vi "MAC BEG.vi"(0 "System no.":i32=1 min=1 max=4 step=1, 2 "Macro name":string, 5 "error in":errorcluster) -> (19 "error out":errorcluster)   [LabVIEW 2026]
doc: "Begin macro recording. Because controller will not answer VI queries during macro recording phase, command VIs cannot be run after this VI to define the macro. Run Define macro contents.vi and finish with MAC END.vi to define a macro.\n\nC-702, C-848, C-867, C-877, C-880, C-884, C-886, C-887, C-891, E-516, E-517, E-518, E-727, E-754, E-816, E-871, E-872, E-873, E-874, F-206,M-8X0, Mercury_GCS: Macro name must be between 1 and 8 characters\n\nE-516: Macro name must be between 3 and 8 characters.Macro will not be saved to FLASH until WPA .vi was run. Changes not saved with WPA are only present in RAM and will be lost when the E-516 is powered off.\n\nE-816: Macro name must be between 3 and 8 characters. Macro will not be saved to FLASH until WPA .vi was run. Changes not saved with WPA are only present in RAM and will be lost when the controller is powered off. This command cannot be issued to a slave. Check controller manual to find out if MAC BEG is supported.\n\nC-887, F-206: Macro name must be between 3 and 8 characters.\n\nMercury: For valid macro names see GCS DLL Manual.\n\nC-887, M-8X0: Macro name must be between 3 and 8 characters. Only for GCS syntax version = GCS 2.0 or higher (check with CSV?.vi. If CSV?.vi is not supported, syntax version is GCS 1.0)."
panel:
  # "Begin macro recording. Because controller will not answer VI\nqueries during macro recording phase, command VIs cannot\nbe run after this VI to define the macro. Run \"Define macro \ncontents.vi\" and finish with \"MAC END.vi\" to define a macro."
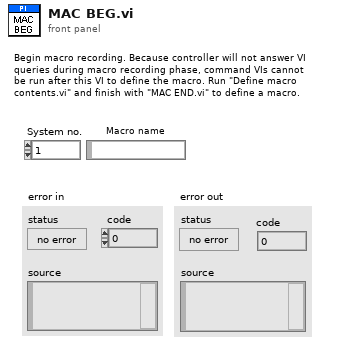
[diagram p1: front panel]
types:
  T1 = enum16{"Disable error check", "Force error check", "Use global settings"}
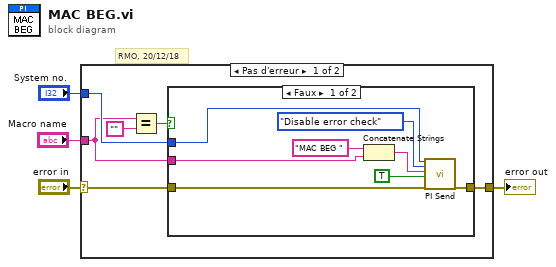
[diagram p0: block diagram]
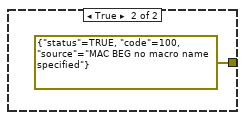
[diagram p2: hidden frame]
diagram:
  # "RMO, 20/12/18"
  n1 = case shown="Pas d'erreur" "error in" {
    selector: "error in" -> [w5 w20]
    tunnel: "System no." -> [w10 _]
    tunnel: [w9 w20] -> w3
    tunnel: "Macro name" -> [w7 _]
    frame No Error {
      n2 = Equal?(x=w7, y="") -> (x = y?=w6:bool)
      n3 = case shown="Faux" w6 {
        tunnel: w5 -> [w18 _]
        tunnel: w10 -> [w15 _]
        tunnel: [w13 errorcluster {"status"=TRUE, "code"=100, "source"="MAC BEG no macro name specified"} ("error out")] -> w9
        tunnel: w7 -> [w12 _]
        frame False {
          n4 = Concatenate Strings("MAC BEG ", w12) -> (w14:string)
          n5 = call "PI Send.vi"("System no."=w15, "Error check settings"=T1."Disable error check", "String to send"=w14, "Attach termination char.?"=TRUE ("Attach Linefeed?"), "error in"=w18) -> ("error out"=w13:errorcluster)  [unwired: 1 in, 13 out]
        }
        frame True {
        }
      }
    }
    frame Error {
    }
  }
  "error out" <- w3
